vi "Copy From IMAQ.vi"() -> ()   [LabVIEW 2020]
uses:
  LabVIEW/g_ar_toolkit.image/g_ar_toolkit.image.lvlib
  LabVIEW/g_ar_toolkit.image/Raw Memory Information Dimension.ctl
  LabVIEW/g_ar_toolkit.image/Raw Memory Information.ctl
  LabVIEW/g_ar_toolkit.image/Image Size (Fixed).ctl
  <vilib>/vision/EDVR.llb/IMAQ ImageToEDVR 2D U32.vi
  LabVIEW/g_ar_toolkit.image/DrawImageToPictureARGB.vi
  LabVIEW/g_ar_toolkit.image/CopyArrayToImageARGB.vi
panel:
  in  "Mode":T1(ring)
  out "IMAQ":T2(plugin-control)
  out "Ouput":picture
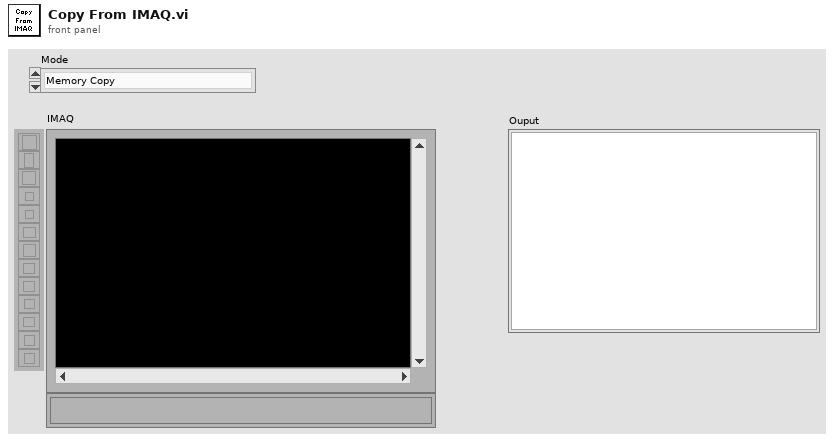
[diagram p1: front panel]
types:
  T1 = enum16{"Memory Copy", "EDVR Access", "Array Values"}
  T2 = typedef "IMAQ Image.ctl" = refnum<image>
  T3 = typedef "Image Type" = u32
  T4 = typedef "g_ar_toolkit.image.lvlib/Image Size (Fixed).ctl" = cluster{"Width":u16, "Height":u16}
  T5 = enum32{"Map Pixel Pointer", "Unmap Pixel Pointer", "Get Pixels Infos"}
  T6 = typedef "g_ar_toolkit.image.lvlib/Raw Memory Information.ctl" = cluster{"Memory Address":u64, "Dimension 0":T7, "Dimension 1":T7}
  T7 = typedef "g_ar_toolkit.image.lvlib/Raw Memory Information Dimension.ctl" = cluster{"Size":u16, "Stride":u32}
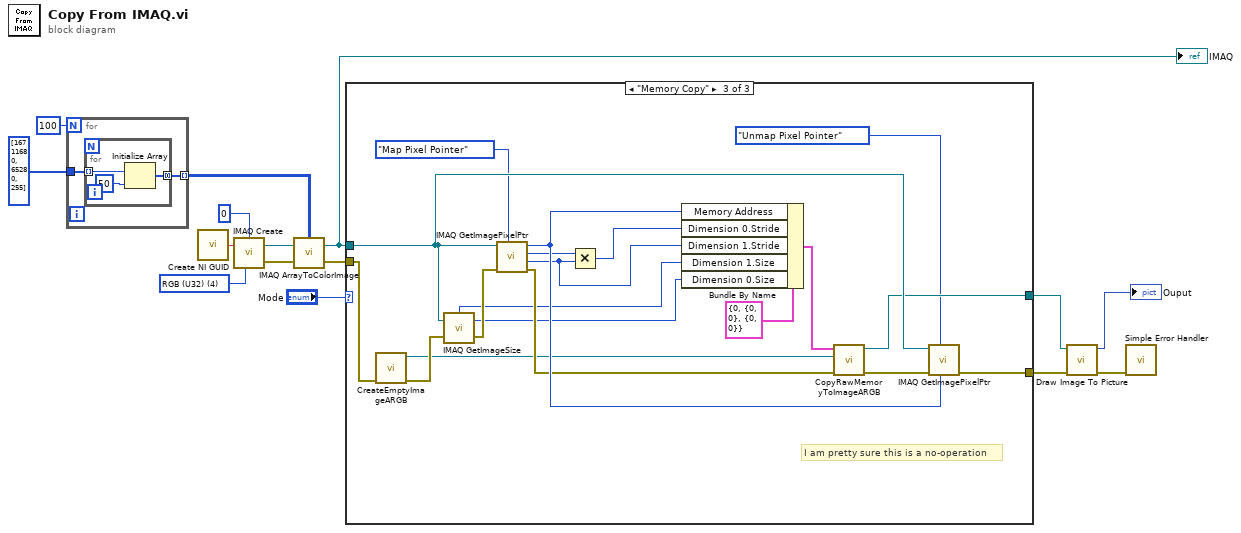
[diagram p0: block diagram]
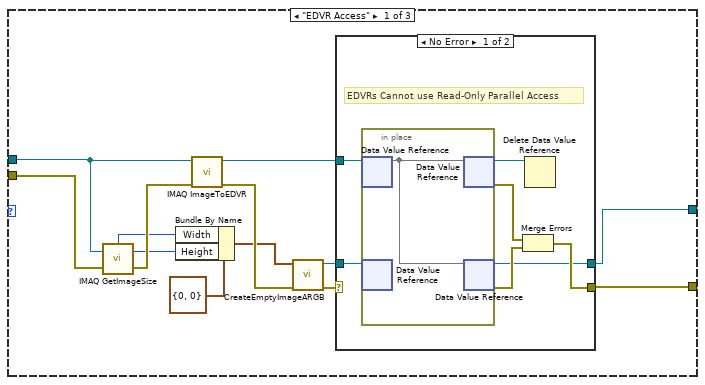
[diagram p2: hidden frame]
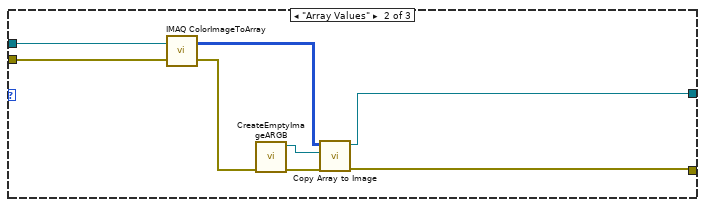
[diagram p4: hidden frame]
diagram:
  w11 = T3 4 items=["Grayscale (U8)", "Grayscale (I16)", "Grayscale (SGL)", "Complex (CSG)", "RGB (U32)", "HSL (U32)", "RGB (U64)", "Grayscale (U16)"] ("Image Type")
  n1 = for {
    N: 100 -> [_]
    tunnel: u32[] [16711680, 65280, 255] ("color(black)") -> [w17]
    tunnel: [w16] -> w12 mode=indexing
    n2 = for {
      tunnel: w17 -> [w20] mode=indexing
      tunnel: [w18] -> w16 mode=concatenating
      n3 = Initialize Array(w20, 50 ("dimension size")) -> (w18:u32[])
    }
  }
  n4 = call <vilib>:"Create NI GUID.vi"() -> ("NI GUID"=w2:string)
  n5 = call "IMAQ Create"("Border Size"=0, "Image Name"=w2, "Image Type"=w11) -> ("New Image"=w15:T2, "error out"=w7:errorcluster)  [unwired: 2 in]
  n6 = call "IMAQ ArrayToColorImage"("Image Pixels (U32)"=w12, "Image"=w15, "error in (no error)"=w7) -> ("Image Out"=w8:T2, "error out"=w10:errorcluster)  [unwired: 2 in]
  "IMAQ" <- w8
  n7 = case shown="\"Memory Copy\"" "Mode" {
    tunnel: w10 -> [w24 w49 w70]
    tunnel: w8 -> [w23 w50 w69]
    tunnel: [w21 w45 w68] -> w6
    tunnel: [w22 w44 w67] -> w5
    frame "EDVR Access" {
      n8 = call "IMAQ GetImageSize"("Image"=w23, "error in (no error)"=w24) -> ("Y Resolution"=w29:i32, "X Resolution"=w28:i32, "error out"=w32:errorcluster)  [unwired: 2 in]
      n9 = Bundle By Name(cluster=T4 {"Width"=0, "Height"=0} ("Preallocated Image Size (Default: 0,0)"), "Width"=w28, "Height"=w29) -> (w30:T4)
      n10 = call-poly <vilib>:"IMAQ ImageToEDVR.vi"("error out"=w32, "Image"=w23) -> ("error out"=w33:errorcluster, "EDVR 2D U32"=w26:refnum<data-value>)  [unwired: 7 in, 1 out]
      n11 = call "CreateEmptyImageARGB.vi"("error in (no error)"=w33, "Preallocated Image Size (Default: 0,0)"=w30) -> ("error out"=w25:errorcluster, "New ARGB Image"=w27:refnum<data-value>)  [unwired: 8 in]
      n12 = case shown="No Error" w25 {
        selector: w25 -> [_ w43]
        tunnel: w27 -> [w40 w42]
        tunnel: w26 -> [w39 _]
        tunnel: [w36 w43] -> w21
        tunnel: [w35 w42] -> w22
        frame No Error {
          # "EDVRs Cannot use Read-Only Parallel Access"
          n13 = in-place {
            n14 = in-place-dvr #1(w39) -> (w41:u32[][])  [unwired: 1 out]
            n15 = in-place-dvr #2(w40) -> ()  [unwired: 2 out]
            n16 = in-place-dvr #1(w41) -> (w34:refnum<data-value>, w37:errorcluster)
            n17 = in-place-dvr #2(w41) -> (w35:refnum<data-value>, w38:errorcluster)
          }
          n18 = Merge Errors(w37, w38) -> (w36:errorcluster)
          n19 = Delete Data Value Reference(data value reference=w34) -> ()  [unwired: 1 in, 2 out]
        }
        frame Error {
        }
      }
    }
    frame "Array Values" {
      n20 = call "IMAQ ColorImageToArray"("Image"=w50, "error in (no error)"=w49) -> ("Image Pixels (U32)"=w46:u32[][], "error out"=w51:errorcluster)  [unwired: 2 in, 1 out]
      n21 = call "CreateEmptyImageARGB.vi"("error in (no error)"=w51) -> ("error out"=w48:errorcluster, "New ARGB Image"=w47:refnum<data-value>)  [unwired: 9 in]
      n22 = call-poly "Copy Array to Image.vi"("error in (no error)"=w48, "ARGB Image Destination"=w47, "Source"=w46) -> ("error out"=w45:errorcluster, "ARGB Image Destination (Duplicate)"=w44:refnum<data-value>)  [unwired: 7 in]
    }
    frame "Memory Copy" {
      # "I am pretty sure this is a no-operation"
      n23 = call "CreateEmptyImageARGB.vi"("error in (no error)"=w70) -> ("error out"=w66:errorcluster, "New ARGB Image"=w52:refnum<data-value>)  [unwired: 9 in]
      n24 = call "IMAQ GetImageSize"("Image"=w69, "error in (no error)"=w66) -> ("Y Resolution"=w55:i32, "X Resolution"=w56:i32, "error out"=w60:errorcluster)  [unwired: 2 in]
      n25 = call "IMAQ GetImagePixelPtr"("Function"=T5."Map Pixel Pointer", "error in (no error)"=w60, "Image"=w69) -> ("error out"=w64:errorcluster, "Pixel Size (Bytes)"=w57:i32, "LineWidth(Pixels)"=w59:i32, "Pixel Pointer out"=w65:u64)  [unwired: 3 in, 2 out]
      n26 = Multiply(x=w59, y=w57) -> (x*y=w58:i32)
      n27 = Bundle By Name(cluster=T6 {"Memory Address"=0, "Dimension 0"={"Size"=0, "Stride"=0}, "Dimension 1"={"Size"=0, "Stride"=0}} ("Source"), "Memory Address"=w65, "Dimension 0.Stride"=w58, "Dimension 1.Stride"=w57, "Dimension 1.Size"=w56, "Dimension 0.Size"=w55) -> (w61:T6)
      n28 = call "CopyRawMemoryToImageARGB.vi"("error in (no error)"=w64, "ARGB Image Destination"=w52, "Source"=w61) -> ("error out"=w54:errorcluster, "ARGB Image Destination (Duplicate)"=w67:refnum<data-value>)  [unwired: 7 in]
      n29 = call "IMAQ GetImagePixelPtr"("Pixel Pointer in"=w65, "Function"=T5."Unmap Pixel Pointer", "error in (no error)"=w54, "Image"=w69) -> ("error out"=w68:errorcluster)  [unwired: 2 in, 5 out]
    }
  }
  n30 = call-poly "Draw Image To Picture.vi"("error in (no error)"=w6, "ARGB Image Source"=w5) -> ("error out"=w3:errorcluster, "Picture"=→"Ouput":picture)  [unwired: 8 in]
  n31 = call <vilib>:"Simple Error Handler.vi"("error in (no error)"=w3) -> ()  [unwired: 4 in, 5 out]
